vi "Add_Props_Marker.vi"(10 "Marker":T2={"Style"=enum."Automatic", "Color"=2147483647, "Size"=0.0} {"Color" items=["Automatic"=2147483647, "Black"=0, "White"=16777215, "Red"=16711680, "Green"=2263842, "Blue"=255, "Cyan"=65535, "Magenta"=16711935, "Yellow"=16776960]}, 11 "Keyword Array":T1[](array[typedef])) -> (3 "Keyword Array Out":T1[](array[typedef]))   [LabVIEW 2013, in "Advanced Plotting Toolkit.lvlib"]
uses:
  Advanced Plotting Toolkit.lvlib
  properties/Marker.ctl
  properties/Marker_Style.ctl
  typedefs/PlotColor.ctl
  KeyValue.ctl
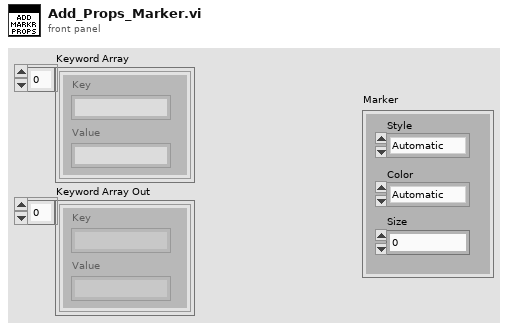
[diagram p1: front panel]
types:
  T1 = typedef "Advanced Plotting Toolkit.lvlib/KeyValue.ctl" = cluster{"Key":string, "Value":string}
  T2 = typedef "Advanced Plotting Toolkit.lvlib/Marker.ctl" = cluster{"Style":T3, "Color":T4, "Size":dbl}
  T3 = typedef "Advanced Plotting Toolkit.lvlib/Marker_Style.ctl" = enum16{"Automatic", "Circle", "Square", "Triangle", "Diamond", "Star", "Invisible"}
  T4 = typedef "Advanced Plotting Toolkit.lvlib/PlotColor.ctl" = u32
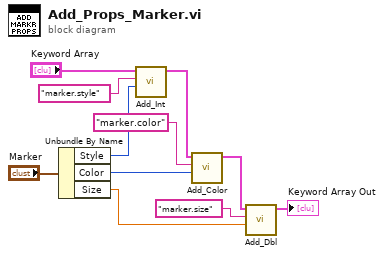
[diagram p0: block diagram]
diagram:
  n1 = Unbundle By Name("Marker") -> ("Style"=w8:T3, "Color"=w5:T4, "Size"=w4:dbl)
  n2 = call "Add_Int.vi"("Value"=w8, "Key"="marker.style", "Keyword Array"="Keyword Array") -> ("Keyword Array Out"=w6:T1[])  [unwired: 8 in]
  n3 = call "Add_Color.vi"("Color"=w5, "Key"="marker.color", "Keyword Array"=w6) -> ("Keyword Array Out"=w3:T1[])  [unwired: 8 in]
  n4 = call "Add_Dbl.vi"("Value"=w4, "Key"="marker.size", "Keyword Array"=w3) -> ("Keyword Array Out"=→"Keyword Array Out":T1[])  [unwired: 8 in]
